vi "Parse Headers.vi"(11 "Raw Header":string) -> (2 "response code":i32, 3 "Parsed Headers":T1[](array[typedef]))   [LabVIEW 2012]
uses:
  Key-Value Pair.ctl
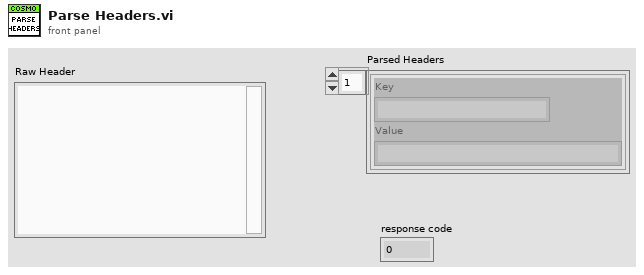
[diagram p1: front panel]
types:
  T1 = typedef "Key-Value Pair.ctl" = cluster{"Key":string, "Value":string}
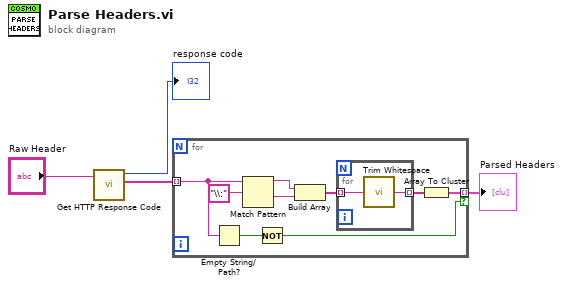
[diagram p0: block diagram]
diagram:
  n1 = call "Get HTTP Response Code.vi"("Header"="Raw Header") -> ("Additional header rows"=w3:string[], "Response code"=→"response code":i32)  [unwired: 8 in, 1 out]
  n2 = for {
    tunnel: w3 -> [w7] mode=indexing
    tunnel: [w13] -> w4 mode=indexing if=w5
    n3 = Empty String/Path?(string/path=w7) -> (empty?=w6:bool)
    n4 = Match Pattern(string=w7, regular expression="\\:") -> (before substring=w9:string, after substring=w8:string)  [unwired: 1 in, 2 out]
    n5 = Not(x=w6) -> (.not. x?=w5:bool)
    n6 = Build Array(w9, w8) -> (w12:string[])
    n7 = for {
      tunnel: w12 -> [w15] mode=indexing
      tunnel: [w14] -> w11 mode=indexing
      n8 = call <vilib>:"Trim Whitespace.vi"("string"=w15) -> ("trimmed string"=w14:string)  [unwired: 1 in]
    }
    n9 = Array To Cluster(array=w11) -> (cluster=w13:cluster{"[0]":string, "[1]":string})
  }
  "Parsed Headers" <- w4
